vi "testArduinoServoPositioning.vi"() -> ()   [LabVIEW 2012]
panel:
  in  "speed":u8
  in  "cancel":bool
  in  "Serial Settings:Baud Rate":u32=57600
  in  "save":bool
  in  "channel":u8
  in  "servo custom position":u16(knob)=1520 max=2500 step=10 scale=0.0..2500.0
  out "error out":errorcluster
  out "serial status":u32(colorbox)=6618880
  in  "VISA resource name":refnum<visa-resource-name>="COM4"
  in  "task":u16(ring) items=["Set custom position", "Enable custom position", "Disable custom position"]
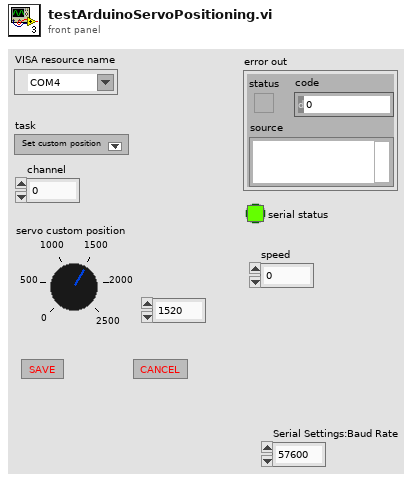
[diagram p1: front panel]
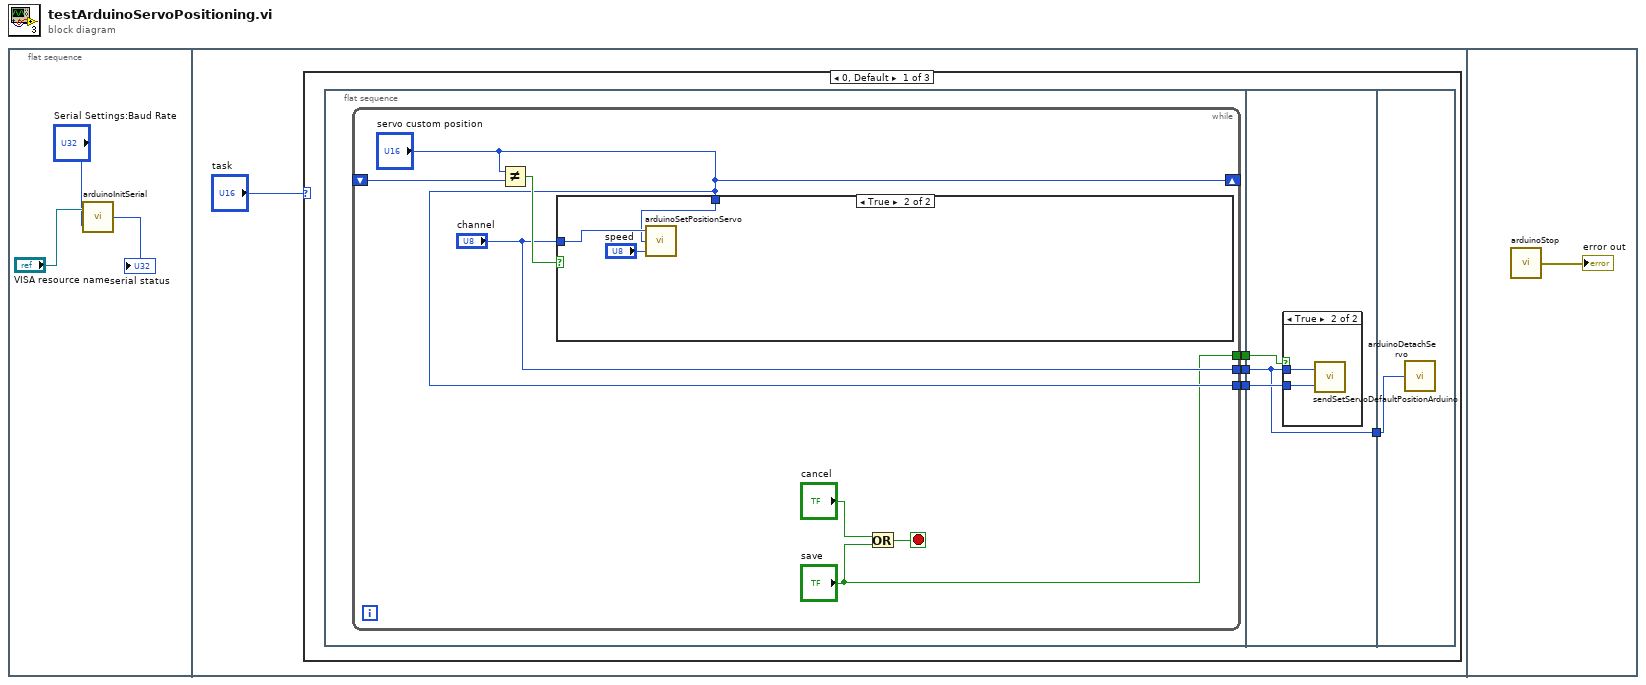
[diagram p0: block diagram]
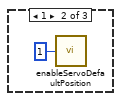
[diagram p4: hidden frame]
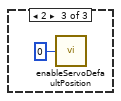
[diagram p5: hidden frame]
diagram:
  n1 = flat-sequence {
    frame #0 {
      n2 = call "arduinoInitSerial.vi"("Serial Settings:Baud Rate"="Serial Settings:Baud Rate", "VISA resource name"="VISA resource name") -> ("serial status"=→"serial status":u32)
    }
    frame #1 {
      n3 = case shown="0, Default" "task" {
        frame 0, Default {
          n4 = flat-sequence {
            tunnel: [w11] -> w8
            tunnel: [w10] -> w7
            tunnel: [w9] -> w6
            tunnel: w8 -> [w22]
            tunnel: w7 -> [w24]
            tunnel: w6 -> [w23]
            tunnel: [w22] -> w5
            tunnel: w5 -> [w27]
            frame #0 {
              n5 = while {
                shift-right: ["servo custom position"] -> _
                shift-left: _ -> [w18]
                tunnel: ["channel"] -> w11
                tunnel: ["servo custom position"] -> w10
                tunnel: ["save"] -> w9
                stop <- w13 stop-if-true
                n6 = Not Equal?(x="servo custom position", y=w18) -> (x != y?=w17:bool)
                n7 = case shown="True" w17 {
                  tunnel: "servo custom position" -> [_ w20]
                  tunnel: "channel" -> [_ w21]
                  frame False {
                  }
                  frame True {
                    n8 = call "arduinoSetPositionServo.vi"("speed"="speed", "servo position"=w20, "channel"=w21) -> ()
                  }
                }
                n9 = Or(x="cancel", y="save") -> (x .or. y?=w13:bool)
              }
            }
            frame #1 {
              n10 = case shown="True" w23 {
                tunnel: w22 -> [_ w26]
                tunnel: w24 -> [_ w25]
                frame False {
                }
                frame True {
                  n11 = call "sendSetServoDefaultPositionArduino.vi"("servo position"=w25, "channel"=w26) -> ()  [unwired: 1 in]
                }
              }
            }
            frame #2 {
              n12 = call "arduinoDetachServo.vi"("channel"=w27) -> ()
            }
          }
        }
        frame 1 {
          n13 = call "enableServoDefaultPosition.vi"("enable bit"=u8 1) -> ()  [unwired: 1 in]
        }
        frame 2 {
          n14 = call "enableServoDefaultPosition.vi"("enable bit"=u8 0) -> ()  [unwired: 1 in]
        }
      }
    }
    frame #2 {
      n15 = call "arduinoStop.vi"() -> ("error out"=→"error out":errorcluster)  [unwired: 2 in]
    }
  }
